vi "9.vi"(11 "文字列":string) -> (3 "検索文字列":string)   [LabVIEW 2019]
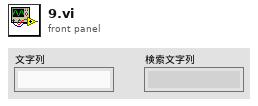
[diagram p1: front panel]
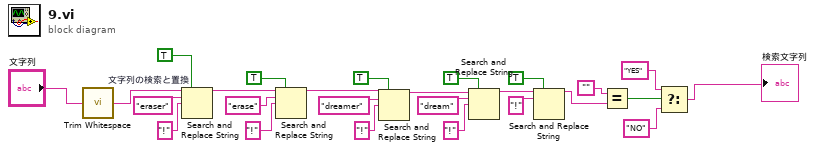
[diagram p0: block diagram]
diagram:
  n1 = call <vilib>:"Trim Whitespace.vi"("string"="文字列") -> ("trimmed string"=w4:string)  [unwired: 1 in]
  n2 = Search and Replace String "文字列の検索と置換"(replace all?=TRUE ("すべて置換? (F)"), input string=w4, search string="eraser" ("検索文字列"), replace string="!" ("置換文字列 (\"\")")) -> (result string=w14:string)  [unwired: 4 in, 3 out]
  n3 = Search and Replace String ("文字列の検索と置換")(replace all?=TRUE ("すべて置換? (F)"), input string=w14, search string="erase" ("検索文字列"), replace string="!" ("置換文字列 (\"\")")) -> (result string=w15:string)  [unwired: 4 in, 3 out]
  n4 = Search and Replace String ("文字列の検索と置換")(replace all?=TRUE ("すべて置換? (F)"), input string=w15, search string="dreamer" ("検索文字列"), replace string="!" ("置換文字列 (\"\")")) -> (result string=w16:string)  [unwired: 4 in, 3 out]
  n5 = Search and Replace String ("文字列の検索と置換")(replace all?=TRUE ("すべて置換? (F)"), input string=w16, search string="dream" ("検索文字列"), replace string="!" ("置換文字列 (\"\")")) -> (result string=w19:string)  [unwired: 4 in, 3 out]
  n6 = Search and Replace String ("文字列の検索と置換")(replace all?=TRUE ("すべて置換? (F)"), input string=w19, search string="!" ("検索文字列")) -> (result string=w21:string)  [unwired: 5 in, 3 out]
  n7 = Equal?(x="", y=w21) -> (x = y?=w22:bool)
  n8 = Select(t="YES" ("検索文字列"), s=w22, f="NO" ("検索文字列")) -> (s? t:f=→"検索文字列":string)
